vi "Load Surface.vi"(8 "error in":errorcluster, 10 "Pixel Format Pointer":u32 format="%.0x", 11 "File":string="c:\\temp\\hello.bmp") -> (0 "error out":errorcluster, 3 "Optimised Surface Pointer":u32 format="%.0x")   [LabVIEW 2015, in "SDL2 Utility.lvlib"]
uses:
  SDL2 Utility.lvlib
  LibSDL2 Wrapper/Controls/NULL.ctl
  LibSDL2 Wrapper/LibSDL2.lvlib
  LibSDL2_Image Wrapper/LibSDL2_Image.lvlib
panel:
  out "Error":string
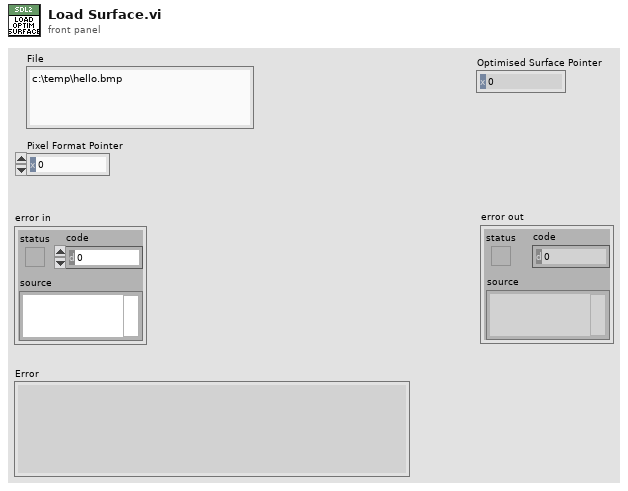
[diagram p1: front panel]
types:
  T1 = typedef "LibSDL2.lvlib/NULL.ctl" = enum32{"NULL"}
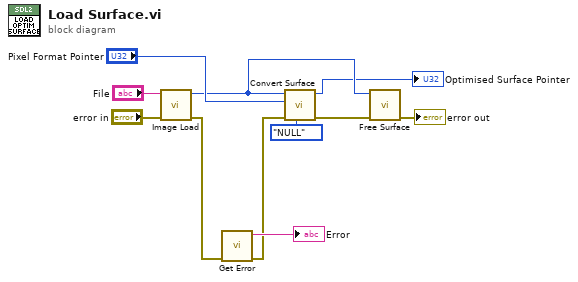
[diagram p0: block diagram]
diagram:
  n1 = call "Image Load.vi"("error in"="error in", "File"="File") -> ("error out"=w2:errorcluster, "Surface Pointer"=w8:u32)  [unwired: 8 in]
  n2 = call "Get Error.vi"("error in"=w2) -> ("error out"=w1:errorcluster, "Error"=→"Error":string)  [unwired: 9 in]
  n3 = call "Convert Surface.vi"("Flags"=NULL."NULL" ("Null"), "error in"=w1, "Pixel Format Pointer"="Pixel Format Pointer", "Loaded Surface Pointer"=w8) -> ("error out"=w5:errorcluster, "Surface Pointer"=→"Optimised Surface Pointer":u32)  [unwired: 6 in]
  n4 = call "Free Surface.vi"("error in"=w5, "Surface Pointer"=w8) -> ("error out"=→"error out":errorcluster)  [unwired: 9 in]
